vi "PushMode.vi"() -> ()   [LabVIEW 2013]
uses:
  PushSubMode.ctl
panel:
  in  "AdjustRate":dbl
  in  "MotorValue":dbl
  in  "SpinRPMChange":dbl
  in  "CurrentRPM":dbl
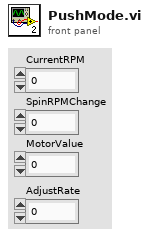
[diagram p1: front panel]
types:
  T1 = typedef "PushSubMode.ctl" = enum16{"Start", "Standby", "Subtract"}
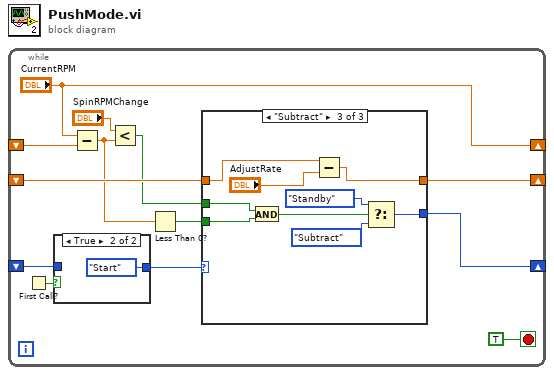
[diagram p0: block diagram]
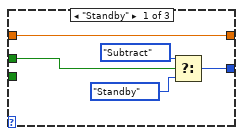
[diagram p3: hidden frame]
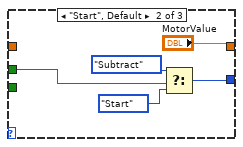
[diagram p4: hidden frame]
diagram:
  n1 = while {
    shift-right: ["CurrentRPM"] -> _
    shift-left: _ -> [w13]
    shift-right: [w11] -> _
    shift-left: _ -> [w10]
    shift-right: [w8] -> _
    shift-left: _ -> [w3]
    stop <- TRUE stop-if-true
    n2 = First Call?() -> (First Call?: T/F=w5:bool)
    n3 = case shown="True" w5 {
      tunnel: [w14 PushSubMode."Start" ("PushSubMode")] -> w4
      tunnel: w3 -> [w14 _]
      frame False {
      }
      frame True {
      }
    }
    n4 = Subtract(x="CurrentRPM", y=w13) -> (x-y=w1:dbl)
    n5 = Less?(x="SpinRPMChange", y=w1) -> (x < y?=w9:bool)
    n6 = Less Than 0?(x=w1) -> (x < 0?=w7:bool)
    n7 = case shown="\"Subtract\"" w4 {
      tunnel: [w20 "MotorValue" w34] -> w11
      tunnel: w10 -> [w20 _ w27]
      tunnel: w9 -> [w16 w22 w30]
      tunnel: [w17 w23 w31] -> w8
      tunnel: w7 -> [_ _ w29]
      frame "Standby" {
        n8 = Select(t=PushSubMode."Subtract" ("PushSubMode"), s=w16, f=PushSubMode."Standby" ("PushSubMode")) -> (s? t:f=w17:T1)
      }
      frame "Start", Default {
        n9 = Select(t=PushSubMode."Subtract" ("PushSubMode"), s=w22, f=PushSubMode."Start" ("PushSubMode")) -> (s? t:f=w23:T1)
      }
      frame "Subtract" {
        n10 = And(x=w30, y=w29) -> (x .and. y?=w28:bool)
        n11 = Subtract(x=w27, y="AdjustRate") -> (x-y=w34:dbl)
        n12 = Select(t=PushSubMode."Standby" ("PushSubMode"), s=w28, f=PushSubMode."Subtract" ("PushSubMode")) -> (s? t:f=w31:T1)
      }
    }
  }
